vi "SINAD Analyzer 1 Chan.vi"(6 "advanced search":T4={"approx freq. (optional)"=-1.0, "search (+/- % of Fsampl.)"=5.0} {"search (+/- % of Fsampl.)" format="%0.2p"; "approx freq. (optional)" format="%0.2p"}, 8 "error in (no error)":errorcluster, 10 "export  mode":T2(ring), 11 "signal in":waveform(dbl)) -> (0 "error out":errorcluster, 1 "THD Plus Noise":dbl format="%.2p", 2 "SINAD (dB)":dbl format="%.2p", 3 "detected fundamental\nfrequency":dbl format="%.2p", 4 "measurement info":T3={"uncertainty"=0.0, "Warning"=FALSE, "comments"="reserved for future use"} {"uncertainty" format="%0.2p"}, 5 "exported signals":T1 {"exported spectrum (dB)"."dB Spectrum (Hann)" format="%.2p"; "exported spectrum (dB)"."df" format="%.2p"; "exported spectrum (dB)"."f0" format="%.2p"})   [LabVIEW 2020, in "NI_MAPro.lvlib"]
doc: "Takes a signal in and performs a full Signal in Noise and Distortion (SINAD) analysis, including measuring the fundamental frequency tone and returning the fundamental frequency and SINAD level in dB. Wire data to the <B>signal in</B> input to determine the polymorphic instance to use or manually select the instance."
uses:
  NI_MAPro.lvlib
  NI_AALBase.lvlib
  NI_MABase.lvlib
panel:
  # "Signal / Noise & Distortion (SINAD) Analyzer"
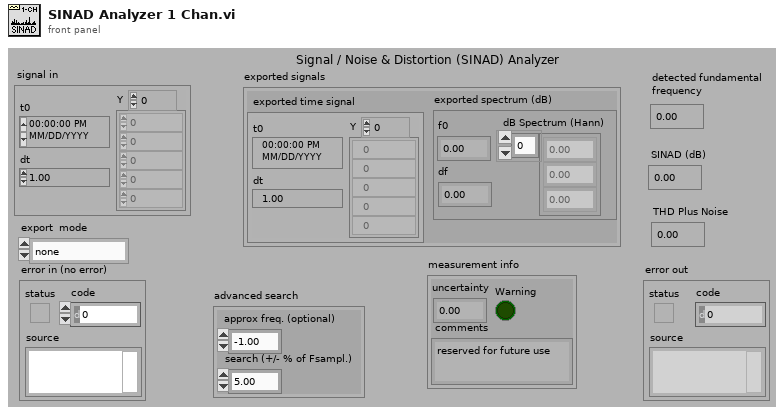
[diagram p1: front panel]
types:
  T1 = cluster{"exported time signal":waveform(dbl), "exported spectrum (dB)":cluster{"f0":dbl, "df":dbl, "dB Spectrum (Hann)":dbl[]}}
  T2 = enum16{"none", "input signal", "fundamental signal", "residual signal"}
  T3 = cluster{"uncertainty":dbl, "Warning":bool, "comments":string}
  T4 = cluster{"approx freq. (optional)":dbl, "search (+/- % of Fsampl.)":dbl}
  T5 = enum16{"none", "input signal", "detected signal", "residual signal"}
  T6 = cluster{"signal in":waveform(dbl), cluster{dbl, dbl, dbl[]}}
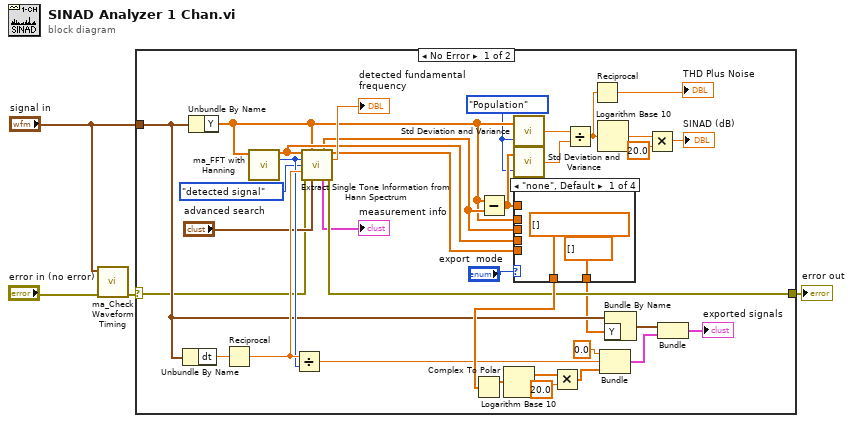
[diagram p0: block diagram]
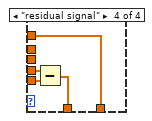
[diagram p4: hidden frame]
diagram:
  n1 = call "ma_Check Waveform Timing.vi"("error in (no error)"="error in (no error)", "signal in"="signal in") -> ("error out"=w3:errorcluster)  [unwired: 1 in, 8 out]
  n2 = case shown="No Error" w3 {
    selector: w3 -> [w5 w50]
    tunnel: [w28 w50] -> w4
    tunnel: "signal in" -> [w15 _]
    frame No Error {
      w8 = enum16{"Sample", "Population"}."Population" ("Weighting (Sample)")
      n3 = Unbundle By Name(w15) -> ("dt"=w16:dbl)
      n4 = Unbundle By Name(w15) -> ("Y"=w17:dbl[])
      n5 = Reciprocal(x=w16) -> (1/x=w32:dbl)
      n6 = call "ma_FFT with Hanning.vi"("time signal data"=w17) -> ("FFT size"=w31:i32, "complex Hann spectrum"=w38:cdb[])  [unwired: 2 in, 7 out]
      n7 = Divide(x=w32, y=w31) -> (x/y=w11:dbl)
      n8 = call "Extract Single Tone Information from Hann Spectrum.vi"("complex spectrum in"=w38, "time signal in"=w17, "FFT size"=w31, "export mode"=T5."detected signal", "sampling frequency"=w32, "error in"=w5, "advanced search"="advanced search") -> ("time signal out"=w27:dbl[], "complex spectrum out"=w37:cdb[], "detected frequency"=→"detected fundamental\nfrequency":dbl, "measurement info"=→"measurement info":T3, "error out"=w28:errorcluster)  [unwired: 4 out]
      n9 = Subtract(x=w17, y=w27) -> (x-y=w26:dbl[])
      n10 = call "Std Deviation and Variance.vi"("X"=w17, "Weighting (Sample)"=w8) -> ("standard deviation"=w22:dbl)  [unwired: 2 out]
      n11 = call "Std Deviation and Variance.vi"("X"=w26, "Weighting (Sample)"=w8) -> ("standard deviation"=w21:dbl)  [unwired: 2 out]
      n12 = case shown="\"none\", Default" "export  mode" {
        tunnel: [dbl[] [] ("Empty array") w43 w45 w46] -> w14
        tunnel: w38 -> [_ w42 _ w49]
        tunnel: w27 -> [_ _ w45 _]
        tunnel: [cdb[] [] ("dB Spectrum (Hann)") w42 w44 w47] -> w36
        tunnel: w17 -> [_ w43 _ _]
        tunnel: w37 -> [_ _ w44 w48]
        tunnel: w26 -> [_ _ _ w46]
        frame "none", Default {
        }
        frame "input signal" {
        }
        frame "fundamental signal" {
        }
        frame "residual signal" {
          n13 = Subtract(x=w49, y=w48) -> (x-y=w47:cdb[])
        }
      }
      n14 = Complex To Polar(r * e^(i*theta)=w36) -> (r=w35:dbl[])  [unwired: 1 out]
      n15 = Logarithm Base 10(1:w35) -> (0:w34:dbl[])
      n16 = Multiply(x=w34, y=20.0) -> (x*y=w12:dbl[])
      n17 = Divide(x=w22, y=w21) -> (x/y=w7:dbl)
      n18 = Reciprocal(x=w7) -> (1/x=→"THD Plus Noise":dbl)
      n19 = Logarithm Base 10(1:w7) -> (0:w20:dbl)
      n20 = Bundle(0.0, w11, w12) -> (w9:cluster{dbl, dbl, dbl[]})  [unwired: 1 out]
      n21 = Bundle By Name(cluster=w15, "Y"=w14) -> (w13:waveform(dbl))
      n22 = Multiply(x=w20, y=20.0) -> (x*y=→"SINAD (dB)":dbl)
      n23 = Bundle("signal in"=w13, w9) -> (→"exported signals":T6)  [unwired: 1 out]
    }
    frame Error {
    }
  }
  "error out" <- w4
